vi "Right Buffer Motion Profile Points.vi"(0 "Motor Name":string, 5 "Time Conversion Factor":dbl=0.48, 7 "Linear Conversion Factor":dbl, 9 "Motion Profile Array":dbl[][](array[numeric]), 11 "PIDF Profile Slot Select":u8) -> (4 "Ready to Execute":bool)   [LabVIEW 2016]
uses:
  <vilib>/Rock Robotics/WPI/ThirdParty/CanMotor/TalonSRX/WPI_CANTalonSRX_APIControlMode.ctl
  <vilib>/Rock Robotics/WPI/ThirdParty/CanMotor/TalonSRX/WPI_CANTalonSRX_GlobalOps.ctl
  <vilib>/Rock Robotics/WPI/ThirdParty/CanMotor/TalonSRX/WPI_CANTalonSRX_MotionProfileTrajectoryPt.ctl
panel:
  out "Initialize Loop Index":i32
  out "Initialize Is Last":bool
  out "Initialize Mot Prof Count":i32
  out "Initialize Mot Prof Buffer Is Full":bool
  out "Total Points in File":i32
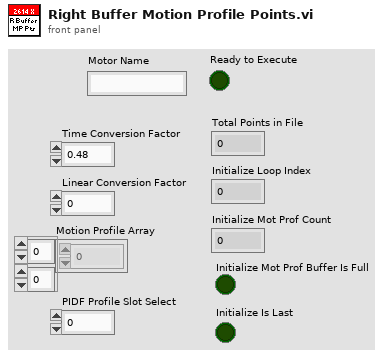
[diagram p1: front panel]
types:
  T1 = typedef "WPI_CANTalonSRX_GlobalOps.ctl" = enum16{"Read For Send", "Write After Receive General", "Write After Receive Feedback", "Write After Receive Encoder", "Write After Receive Ain", "Write Error", "Get All", "Set Output", "Set Mode", "Set Master ID", "Set Brake Mode", "Set Reverse Feedback Sensor", "Set Reverse Closed Loop Output", "Set Override Limits", "Set Forward Limit Enabled", "Set Reverse Limit Enabled", "Set Feedback Select", "Set Profile Select", "Set Throttle Ramp Rate", "Disable", "Set Enc Codes Per Rev", "Set Num Pot Turns", "Set Control Frame Rate", "Enable Legacy Control", "Write After Receive Pulse Width", "Set Enable Frame Rate", "Write After Receive Motion Profile", "Set Motion Profile Flow Control", "Set Motion Profile Control Frame Rate", "Set Current Limit Enable"}
  T2 = typedef "WPI_CANTalonSRX_APIControlMode.ctl" = enum8{"Percent VBus", "Speed", "Position", "Slave", "Unchanged / Invalid", "Voltage Compensation", "Current", "Motion Profile", "Motion Magic"}
  T3 = typedef "WPI_MotorControlDeviceRef.ctl" = cluster{"DeviceStatus":errorcluster, "Type":T4, "PWM":cluster{"PWM Channel":T5, "DeadBand":T6}, "CAN":cluster{"Device Number":u8, "SetOutput VI Ref":variant, "GetOutput VI Ref":variant, "Enable VI Ref":variant, "Disable VI Ref":variant, "Data":variant}, "Invert":bool}
  T4 = typedef "WPI_MotorControlType.ctl" = enum16{"PWM", "CAN"}
  T5 = typedef "FPGA_DIOPWMChannel.ctl" = enum8{"PWM 0", "PWM 1", "PWM 2", "PWM 3", "PWM 4", "PWM 5", "PWM 6", "PWM 7", "PWM 8", "PWM 9", "PWM MXP 0", "PWM MXP 1", "PWM MXP 2", "PWM MXP 3", "PWM MXP 4", "PWM MXP 5", "PWM MXP 6", "PWM MXP 7", "PWM MXP 8", "PWM MXP 9", "Invalid"}
  T6 = typedef "WPI_PWMDeadband.ctl" = cluster{"Name":string, "maxPositivePwm":i32, "minPositivePwm":i32, "centerPwm":i32, "maxNegativePwm":i32, "minNegativePwm":i32, "angularRange":u16}
  T7 = typedef "WPI_CANTalonSRX_MotionProfileTrajectoryPt.ctl" = cluster{"Duration Ms":u8, "Velocity":dbl, "Position":dbl, "Profile Slot Select":u8, "Is Last":bool, "Velocity Only":bool, "Zero Position":bool, "Compress Code":u8, "Same Velocity":i32, "Delta Position":i32, "Count":u8}
  T8 = typedef "WPI_CANTalonSRX_GlobalStatus.ctl" = cluster{"Applied Throttle":dbl, "Module Enabled":bool, "CAN Error":errorcluster, "Closed Loop Error":dbl, "Forward Limit Switch Closed":bool, "Reverse Limit Switch Closed":bool, "Sensor Position":dbl, "Sensor Velocity":dbl, "Current":dbl, "Sticky Fault - Over Temp":bool, "Sticky Fault - Under Voltage":bool, "Sticky Fault - Forward Limit":bool, "Sticky Fault - Reverse Limit":bool, "Sticky Fault - Forward Soft Limit":bool, "Sticky Fault - Reverse Soft Limit":bool, "Brake is Enabled":bool, "Encoder Position":dbl, "Encoder Velocity":dbl, "Encoder Index Count":dbl, "Encoder A Pin State":bool, "Encoder B Pin State":bool, "Encoder Index Pin State":bool, "Analog In":dbl, "Analog In Velocity":dbl, "Temperature (C)":dbl, "Battery Voltage":dbl, "Control 5 Is Supported":bool, "Current Profile Slot Select":dbl, "Pos Div 8":bool, "Vel Div 4":bool, "Pulse Width Position":i32, "Pulse Width Velocity":i32, "Pulse Width Rise To Rise (us)":i32, "Pulse Width Rise To Fall (us)":i32, "Mot Prof Active Is Under Run":bool, "Mot Prof Active Has Under Run":bool, "Mot Prof Active Is Last":bool, "Mot Prof Active Velocity Only":bool, "Mot Prof Active Is Valid":bool, "Mot Prof Buffer Is Full":bool, "Mot Prof Active Profile Slot Select":i32, "Mot Prof NextID":i32, "Mot Prof Count":i32, "Mot Prof Active Velocity":dbl, "Mot Prof Active Position":dbl, "Mot Prof Output Enable":i32}
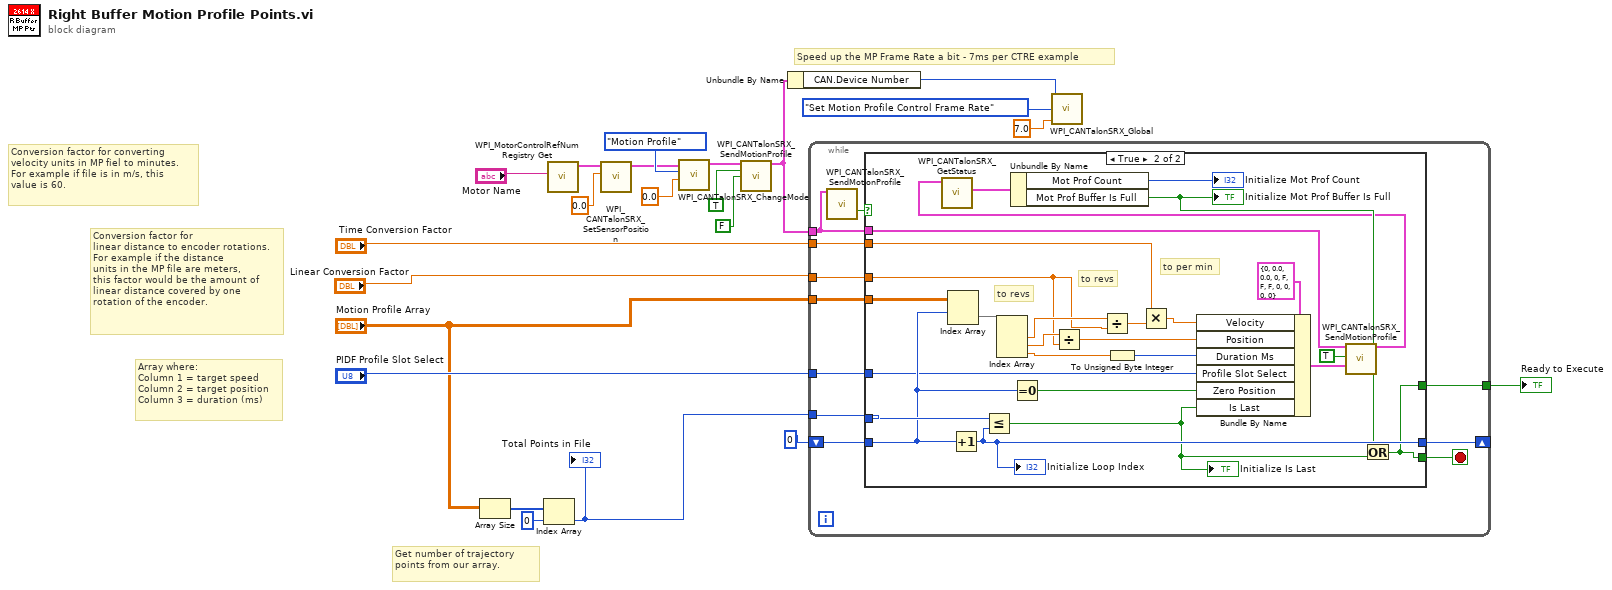
[diagram p0: block diagram]
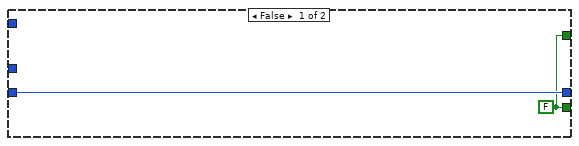
[diagram p2: hidden frame]
diagram:
  # "Array where:\nColumn 1 = target speed\nColumn 2 = target position\nColumn 3 = duration (ms)"
  # "Conversion factor for converting \nvelocity units in MP fiel to minutes.\nFor example if file is in m/s, this\nvalue is 60."
  # "Conversion factor for\nlinear distance to encoder rotations.\nFor example if the distance\nunits in the MP file are meters,\nthis factor would be the amount of\nlinear distance covered by one\nrotation of the encoder."
  # "Speed up the MP Frame Rate a bit - 7ms per CTRE example"
  # "Get number of trajectory points from our array."
  n1 = Array Size(array="Motion Profile Array") -> (size(s)=w17:i32[])
  n2 = Index Array(array=w17, index=0) -> (element=w12:i32)
  "Total Points in File" <- w12
  n3 = call <vilib>:"WPI_MotorControlRefNum Registry Get.vi"("refnum name"="Motor Name") -> ("MotorControlDevRef"=w22:T3)  [unwired: 9 in, 1 out]
  n4 = call <vilib>:"WPI_CANTalonSRX_SetSensorPosition.vi"("New Sensor Position"=0.0, "CAN Talon SRX Ref"=w22) -> ("CAN Talon SRX Ref"=w18:T3)  [unwired: 8 in, 1 out]
  n5 = call <vilib>:"WPI_CANTalonSRX_ChangeMode.vi"("Output"=0.0, "Control Mode"=WPI_CANTalonSRX_APIControlMode."Motion Profile", "CAN Talon SRX Ref"=w18) -> ("CAN Talon SRX Ref"=w15:T3)  [unwired: 7 in, 1 out]
  n6 = call <vilib>:"WPI_CANTalonSRX_SendMotionProfile.vi"("CAN Talon SRX Ref"=w15, "Clear"=TRUE, "Push"=FALSE) -> ("CAN Talon SRX Ref Out"=w10:T3)  [unwired: 9 in, 3 out]
  n7 = Unbundle By Name(w10) -> ("CAN.Device Number"=w9:u8)
  n8 = while {
    tunnel: w10 -> [w26]
    shift-right: [w32] -> _
    shift-left: 0 -> [w30]
    tunnel: w12 -> [w33]
    tunnel: "Motion Profile Array" -> [w31]
    tunnel: "Linear Conversion Factor" -> [w29]
    tunnel: "Time Conversion Factor" -> [w28]
    tunnel: "PIDF Profile Slot Select" -> [w27]
    tunnel: [w23] -> w2
    stop <- w24 stop-if-true
    n9 = call <vilib>:"WPI_CANTalonSRX_SendMotionProfile.vi"("CAN Talon SRX Ref"=w26) -> ("Ready For Next"=w25:bool)  [unwired: 11 in, 3 out]
    n10 = case shown="True" w25 {
      tunnel: w33 -> [_ w61]
      tunnel: [w35 w60] -> w32
      tunnel: w31 -> [_ w54]
      tunnel: w30 -> [w35 w53]
      tunnel: w29 -> [_ w50]
      tunnel: w28 -> [_ w43]
      tunnel: w27 -> [_ w42]
      tunnel: w26 -> [_ w40]
      tunnel: [w34 w38] -> w24
      tunnel: [w34 w38] -> w23
      frame False {
        w34 = FALSE
      }
      frame True {
        # "to per min"
        # "to revs"
        # "to revs"
        n11 = Index Array(array=w54, index (row)=w53) -> (element=w55:dbl[])  [unwired: 1 in]
        n12 = Increment(x=w53) -> (x+1=w60:i32)
        "Initialize Loop Index" <- w60
        n13 = Less Or Equal?(x=w61, y=w60) -> (x <= y?=w36:bool)
        "Initialize Is Last" <- w36
        n14 = Index Array(array=w55) -> (element #1=w52:dbl, element #2=w51:dbl, element #3=w45:dbl)  [unwired: 3 in]
        n15 = Equal To 0?(x=w53) -> (x = 0?=w57:bool)
        n16 = Divide(x=w51, y=w50) -> (x/y=w47:dbl)
        n17 = Divide(x=w52, y=w50) -> (x/y=w49:dbl)
        n18 = To Unsigned Byte Integer(number=w45) -> (unsigned 8bit integer=w44:u8)
        n19 = Multiply(x=w43, y=w49) -> (x*y=w48:dbl)
        n20 = Bundle By Name(cluster=T7 {"Duration Ms"=0, "Velocity"=0.0, "Position"=0.0, "Profile Slot Select"=0, "Is Last"=FALSE, "Velocity Only"=FALSE, "Zero Position"=FALSE, "Compress Code"=0, "Same Velocity"=0, "Delta Position"=0, "Count"=0} ("New Point"), "Velocity"=w48, "Position"=w47, "Duration Ms"=w44, "Profile Slot Select"=w42, "Zero Position"=w57, "Is Last"=w36) -> (w58:T7)
        n21 = call <vilib>:"WPI_CANTalonSRX_SendMotionProfile.vi"("CAN Talon SRX Ref"=w40, "Push"=TRUE, "New Point"=w58) -> ("CAN Talon SRX Ref Out"=w37:T3)  [unwired: 9 in, 3 out]
        n22 = call <vilib>:"WPI_CANTalonSRX_GetStatus.vi"("CAN Talon SRX Ref"=w37) -> ("Talon SRX Status"=w46:T8)  [unwired: 8 in, 2 out]
        n23 = Unbundle By Name(w46) -> ("Mot Prof Count"=→"Initialize Mot Prof Count":i32, "Mot Prof Buffer Is Full"=w39:bool)
        "Initialize Mot Prof Buffer Is Full" <- w39
        n24 = Or(x=w39, y=w36) -> (x .or. y?=w38:bool)
      }
    }
  }
  "Ready to Execute" <- w2
  n25 = call <vilib>:"WPI_CANTalonSRX_Global.vi"("Set Number"=7.0, "Operation"=WPI_CANTalonSRX_GlobalOps."Set Motion Profile Control Frame Rate", "Device ID (0)"=w9) -> ()  [unwired: 6 in, 3 out]
